vi "Stop.vi"(8 "error in (no error)":errorcluster, 11 "User Interface Handler in":refnum<class "User Interface Handler.lvclass">) -> (0 "error out":errorcluster, 3 "User Interface Handler out":refnum<class "User Interface Handler.lvclass">)   [LabVIEW 2020, in "DSF Core.lvlib" / "User Interface Handler.lvclass"]
uses:
  User Interface Handler.lvclass
  User Interface Handler.lvclass/User Interface Handler.ctl
  User Interface Events/User Interface Events.lvclass
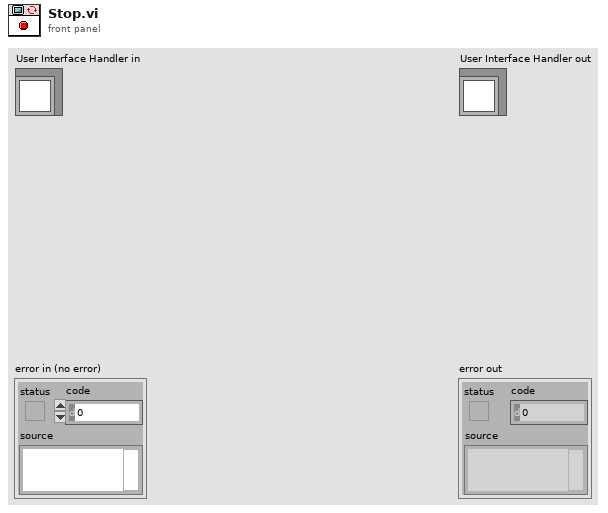
[diagram p1: front panel]
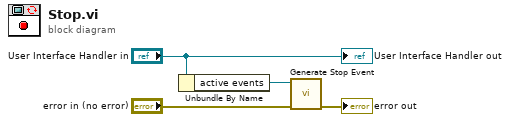
[diagram p0: block diagram]
diagram:
  n1 = Unbundle By Name("User Interface Handler in") -> ("active events"=w3:refnum<class "User Interface Events.lvclass">)
  n2 = call "Generate Stop Event.vi"("error in (no error)"="error in (no error)", "User Interface Events in"=w3) -> ("error out"=→"error out":errorcluster)  [unwired: 8 in, 1 out]
  "User Interface Handler out" <- "User Interface Handler in"
